vi "Unsigned In Range and Coerce.vi"(9 "Lower Limit":dbl, 10 "Input":dbl, 11 "Upper Limit":dbl) -> (2 "Output":dbl)   [LabVIEW 2013]
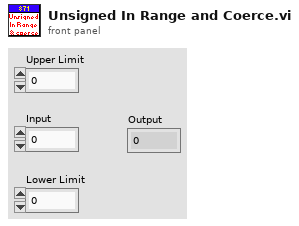
[diagram p1: front panel]
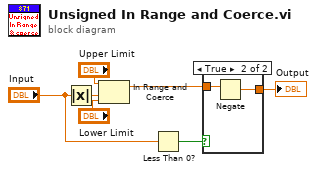
[diagram p0: block diagram]
diagram:
  n1 = Absolute Value(x="Input") -> (abs(x)=w7:dbl)
  n2 = In Range and Coerce(upper limit="Upper Limit", x=w7, lower limit="Lower Limit") -> (coerced(x)=w2:dbl)  [unwired: 1 out]
  n3 = Less Than 0?(x="Input") -> (x < 0?=w3:bool)
  n4 = case shown="True" w3 {
    tunnel: w2 -> [w8 w10]
    tunnel: [w8 w9] -> w1
    frame False {
    }
    frame True {
      n5 = Negate(x=w10) -> (-x=w9:dbl)
    }
  }
  "Output" <- w1
